vi "MedianFilter_Calculate.vi"(9 "Input Value":dbl, 11 "In MEDIAN_FILTER":T1 {"ValueBuffer" format="%13.5g"}) -> (1 "MedianValue":dbl, 3 "Out MEDIAN_FILTER":T1 {"ValueBuffer" format="%13.5g"})   [LabVIEW 2019, in "Trajectory_Library.lvlib"]
doc: "Calculates the moving-window median for the next value of the input stream.\n\nInputs:\n - In Median Filter -- Median filter data structure\n - Input Value -- The next input value. \n\nOutputs:\n - Out Median Filter -- Updated median filter data structure\n - Median Value -- The median of the moving window, updated to include the next value.."
uses:
  Trajectory_Library.lvlib
  <vilib>/Analysis/NI_AALBase.lvlib
  TypeDef/MEDIAN_FILTER.ctl
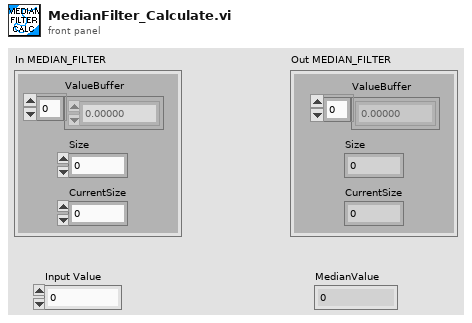
[diagram p1: front panel]
types:
  T1 = typedef "Trajectory_Library.lvlib/MEDIAN_FILTER.ctl" = cluster{"ValueBuffer":dbl[], "Size":i32, "CurrentSize":i32}
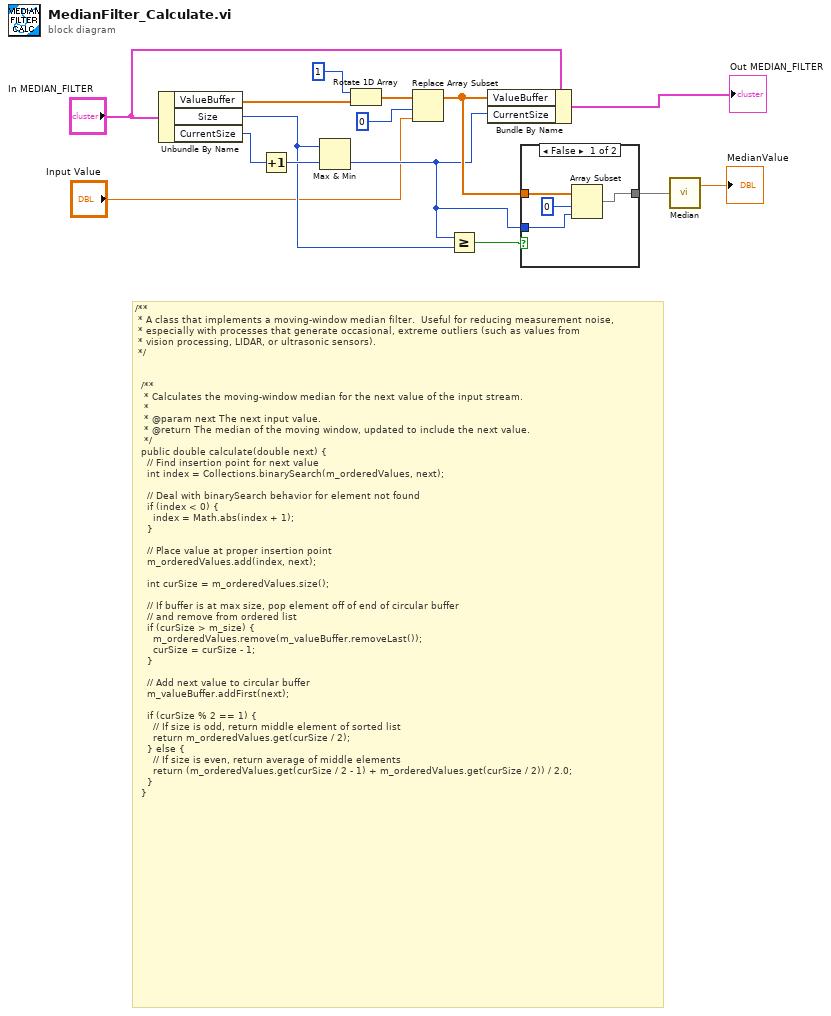
[diagram p0: block diagram]
diagram:
  # "/**\n * A class that implements a moving-window median filter.  Useful for reducing measurement noise,\n * especially with processes that generate occasional, extreme outliers (such as values from\n * vision processing, LIDAR, or ultrasonic sensors).\n */\n\n\n  /**\n   * Calculates the moving-window median for the next value of the input stream.\n   *\n   * @param next The next input value.\n   * @return The median of the moving window, updated to include the next value.\n   */\n  public double calculate(double next) {\n    // Find insertion point for next value\n    int index = Collections.binarySearch(m_orderedValues, next);\n\n    // Deal with binarySearch behavior for element not found\n    if (index < 0) {\n      index = Math.abs(index + 1);\n    }\n\n    // Place value at proper insertion point\n    m_orderedValues.add(index, next);\n\n    int curSize = m_orderedValues.size();\n\n    // If buffer is at max size, pop element off of end of circular buffer\n    // and remove from ordered list\n    if (curSize > m_size) {\n      m_orderedValues.remove(m_valueBuffer.removeLast());\n      curSize = curSize - 1;\n    }\n\n    // Add next value to circular buffer\n    m_valueBuffer.addFirst(next);\n\n    if (curSize % 2 == 1) {\n      // If size is odd, return middle element of sorted list\n      return m_orderedValues.get(curSize / 2);\n    } else {\n      // If size is even, return average of middle elements\n      return (m_orderedValues.get(curSize / 2 - 1) + m_orderedValues.get(curSize / 2)) / 2.0;\n    }\n  }"
  n1 = Unbundle By Name("In MEDIAN_FILTER") -> ("ValueBuffer"=w15:dbl[], "Size"=w7:i32, "CurrentSize"=w11:i32)
  n2 = Increment(x=w11) -> (x+1=w10:i32)
  n3 = Max & Min(x=w7, y=w10) -> (min(x,y)=w6:i32)  [unwired: 1 out]
  n4 = Rotate 1D Array(1:w15, 2:1 ("n")) -> (0:w14:dbl[])
  n5 = Replace Array Subset(array=w14, new element="Input Value", index=0) -> (w9:dbl[])
  n6 = Greater Or Equal?(x=w6, y=w7) -> (x >= y?=w5:bool)
  n7 = Bundle By Name(cluster="In MEDIAN_FILTER", "ValueBuffer"=w9, "CurrentSize"=w6) -> (→"Out MEDIAN_FILTER":T1)
  n8 = case shown="False" w5 {
    tunnel: w9 -> [w18 w20]
    tunnel: [w16 w20] -> w8
    tunnel: w6 -> [w17 _]
    frame False {
      n9 = Array Subset(array=w18, index=0, length=w17) -> (w16:dbl[])
    }
    frame True {
    }
  }
  n10 = call <vilib>:"Median.vi"("X"=w8) -> ("median"=→"MedianValue":dbl)  [unwired: 1 out]
